vi "Write ConnectAct.vi"(8 "error in (no error)":errorcluster, 10 "ConnectAct?":bool, 11 "IOCard in":refnum<class "IOCard.lvclass">) -> (0 "error out":errorcluster, 3 "IOCard out":refnum<class "IOCard.lvclass">)   [LabVIEW 2019]
uses:
  IOCard.lvclass
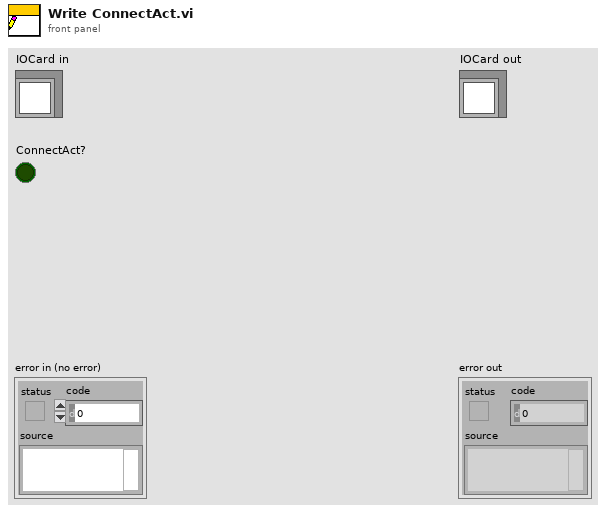
[diagram p1: front panel]
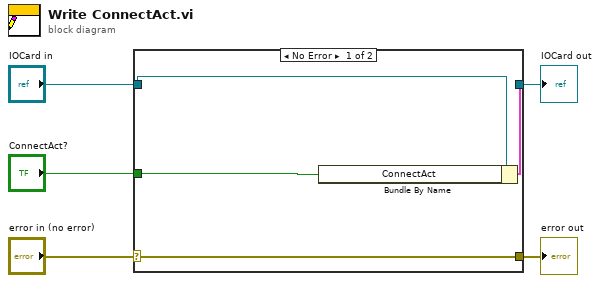
[diagram p0: block diagram]
diagram:
  n1 = case shown="No Error" "error in (no error)" {
    selector: "error in (no error)" -> [w9 w10]
    tunnel: [w9 w10] -> w4
    tunnel: [w7 w11] -> w2
    tunnel: "IOCard in" -> [w8 w11]
    tunnel: "ConnectAct?" -> [w6 _]
    frame No Error {
      n2 = Bundle By Name(cluster=w8, "ConnectAct"=w6) -> (w7:cluster{})
    }
    frame Error {
    }
  }
  "error out" <- w4
  "IOCard out" <- w2
